vi "Bob Recreate Quantum Key.vi"(8 "error in":errorcluster, 10 "Correct Measurements Indexes in":u32[](array[numeric]), 11 "Raw Data in":u8[](array[numeric])) -> (0 "error out":errorcluster, 1 "Incorrect Alice's data":bool, 2 "Sifted Key out":u8[](array[numeric]))   [LabVIEW 2018]
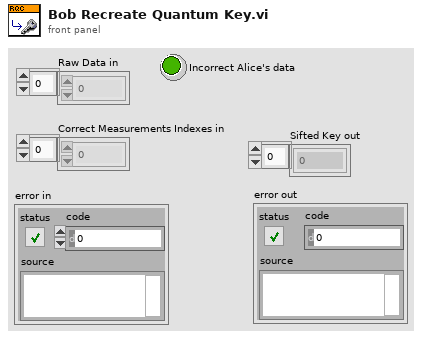
[diagram p1: front panel]
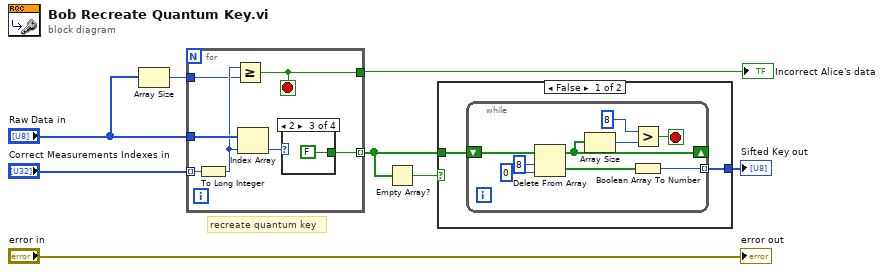
[diagram p0: block diagram]
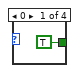
[diagram p3: hidden frame]
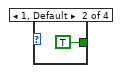
[diagram p4: hidden frame]
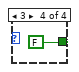
[diagram p5: hidden frame]
diagram:
  # "recreate quantum key"
  n1 = Array Size(array="Raw Data in") -> (size(s)=w7:i32)
  n2 = for {
    tunnel: "Raw Data in" -> [w15]
    tunnel: "Correct Measurements Indexes in" -> [w14] mode=indexing
    tunnel: w7 -> [w12]
    tunnel: [w11] -> w5
    tunnel: [w9] -> w1 mode=indexing
    stop <- w11 stop-if-true
    n3 = To Long Integer(number=w14) -> (32bit integer=w13:i32)
    n4 = Greater Or Equal?(x=w13, y=w12) -> (x >= y?=w11:bool)
    n5 = Index Array(array=w15, index=w13) -> (element=w10:u8)
    n6 = case shown="2" w10 {
      tunnel: [TRUE TRUE FALSE FALSE] -> w9
      frame 0 {
      }
      frame 1, Default {
      }
      frame 2 {
      }
      frame 3 {
      }
    }
  }
  "Incorrect Alice's data" <- w5
  n7 = Empty Array?(array=w1) -> (empty?=w2:bool)
  n8 = case shown="False" w2 {
    tunnel: w1 -> [w21 _]
    tunnel: [w20 _] -> w4
    frame False {
      n9 = while {
        shift-right: [w24] -> _
        shift-left: w21 -> [w30]
        tunnel: [w25] -> w20 mode=indexing
        stop <- w29 stop-if-true
        n10 = Delete From Array(array=w30, length=8, index=0) -> (deleted portion=w26:bool[], array with subset deleted=w24:bool[])
        n11 = Array Size(array=w24) -> (size(s)=w23:i32)
        n12 = Greater?(x=8, y=w23) -> (0:w29:bool)
        n13 = Boolean Array To Number(Boolean array=w26) -> (number=w25:u8)
      }
    }
    frame True {
    }
  }
  "Sifted Key out" <- w4
  "error out" <- "error in"
